vi "TestVariantConverstions.vi"() -> ()   [LabVIEW 2017]
panel:
  out "After":cluster{"Numeric":dbl}[](array[cluster])
  out "Array as variant":variant
  out "As variant array":variant[](array[variant])
  in  "PadBy":dbl
  in  "TesyClusterArray":cluster{"Numeric":dbl}[](array[cluster])
  out "Totallength":u32
  out "data":dbl[](array[numeric])
  in  "Numeric":dbl[][](array[numeric])
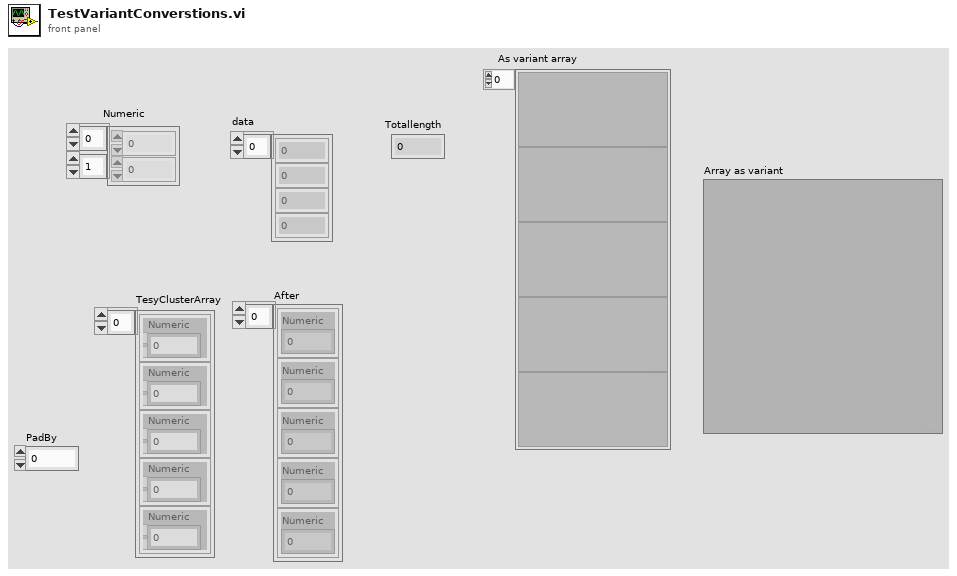
[diagram p1: front panel]
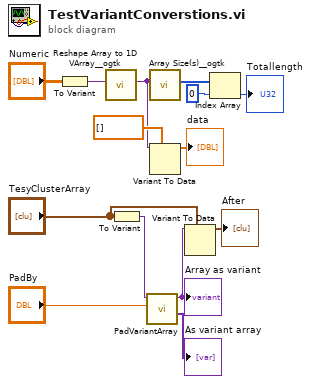
[diagram p0: block diagram]
diagram:
  n1 = To Variant(anything="Numeric") -> (Variant=w13:variant)
  n2 = call <userlib>:"Reshape Array to 1D VArray__ogtk.vi"("MultiD Array"=w13) -> ("1D VArray"=w7:variant)  [unwired: 8 in, 2 out]
  n3 = To Variant(anything="TesyClusterArray") -> (Variant=w6:variant)
  n4 = call "PadVariantArray.vi"("PadBy"="PadBy", "Array In"=w6) -> ("Array of variant values"=→"As variant array":variant[], "Array out"=w2:variant)  [unwired: 8 in]
  "Array as variant" <- w2
  n5 = call <userlib>:"Array Size(s)__ogtk.vi"("Array"=w7) -> ("Size(s)"=w10:u32[])  [unwired: 8 in, 2 out]
  n6 = Variant To Data(type=dbl[] [], Variant=w7) -> (data=→"data":dbl[])  [unwired: 1 in, 1 out]
  n7 = Variant To Data(type="TesyClusterArray", Variant=w2) -> (data=→"After":cluster{"Numeric":dbl}[])  [unwired: 1 in, 1 out]
  n8 = Index Array(array=w10, index=0) -> (element=→"Totallength":u32)
